vi "Verify Font availability.vi"(0 "Font IN":refnum<class "Font Class.lvclass">, 7 "Font name":string, 9 "One button message (F)?":bool, 11 "error in (no error)":errorcluster) -> (4 "Font duplicate":refnum<class "Font Class.lvclass">, 8 "Font":string, 15 "error out":errorcluster)   [LabVIEW 2019, in "Exaprom PDF.lvlib" / "Font Class.lvclass"]
doc: "Version 1.0\nDeveloped by Jean-Marc Simard\nCopyright © 2010, Exaprom Inc.\nAll rights reserved.\nLicense: BSD\n\nWith iTextSharp 4.1.6 (http://itextsharp.sourceforge.net)\nunder Mozilla Public License Version 1.1\n(http://www.mozilla.org/MPL/MPL-1.1.html)"
uses:
  Font Class.lvclass
  Font Class.lvclass/Font Class.ctl
  Exaprom PDF.lvlib
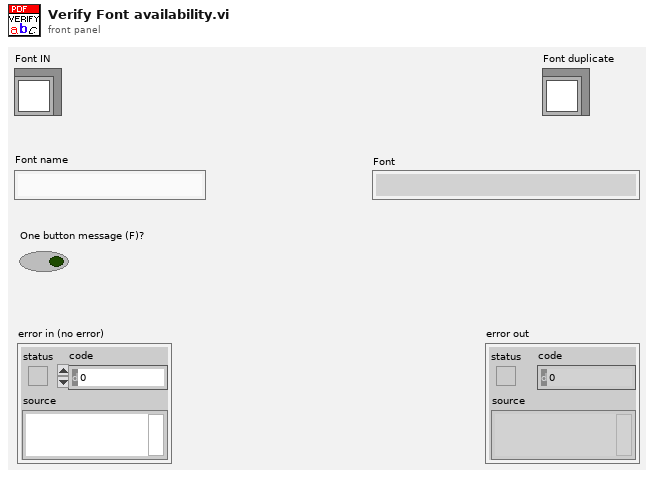
[diagram p1: front panel]
types:
  T1 = cluster{"Font name":string, "File name":string}[]
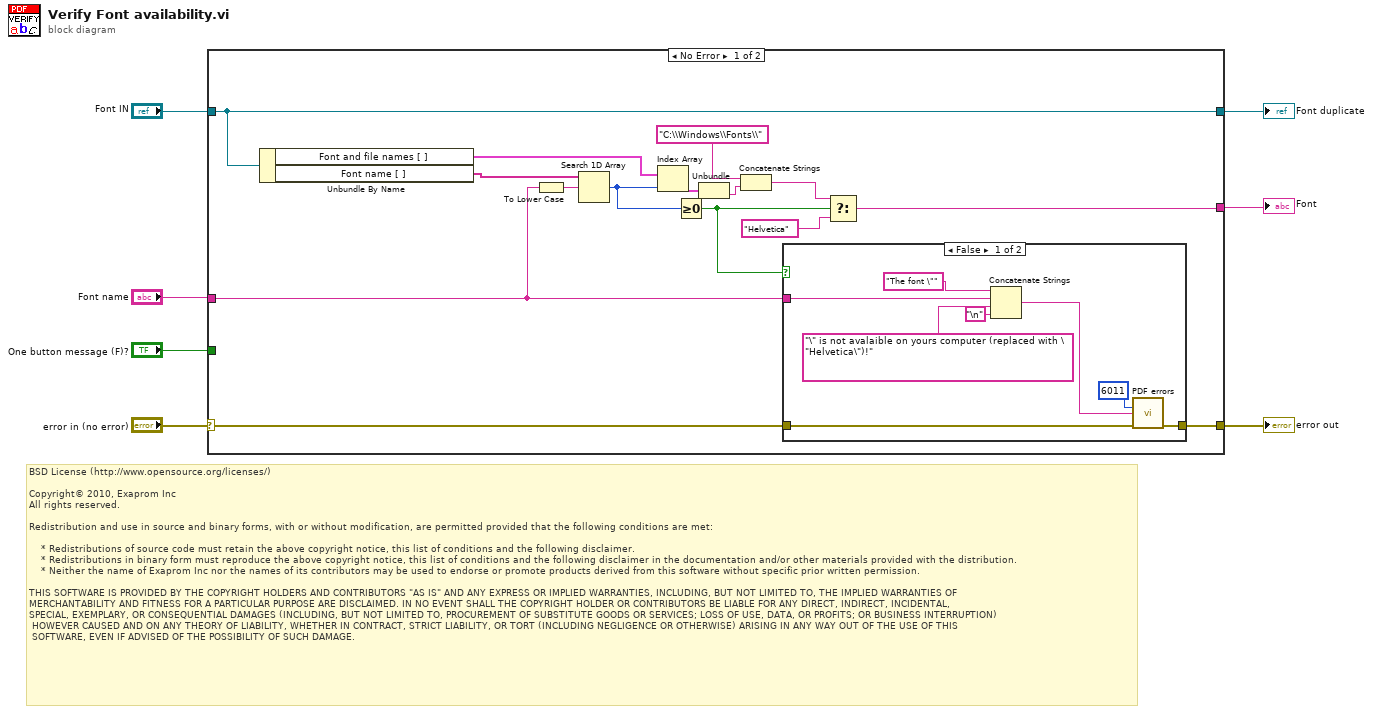
[diagram p0: block diagram]
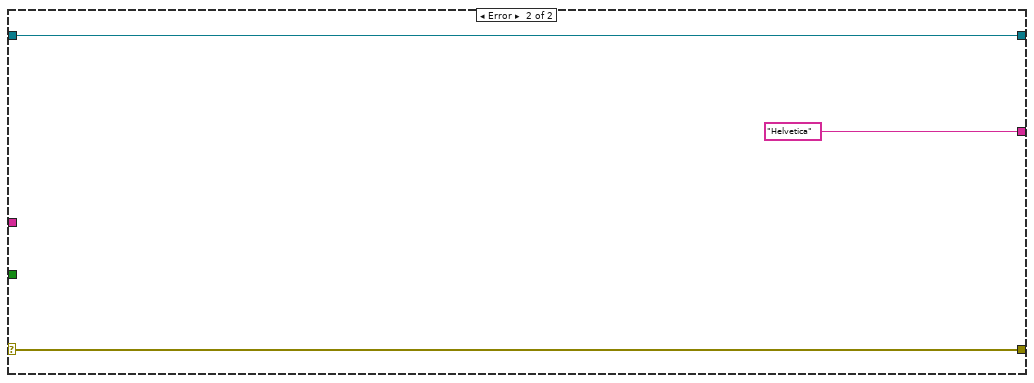
[diagram p3: hidden frame]
diagram:
  # "BSD License (http://www.opensource.org/licenses/)\n\nCopyright© 2010, Exaprom Inc\nAll rights reserved.\n\nRedistribution and use in source and binary forms, with or without modification, are permitted provided that the following conditions are met:\n\n    * Redistributions of source code must retain the above copyright notice, this list of conditions and the following disclaimer.\n    * Redistributions in binary form must reproduce the above copyright notice, this list of conditions and the following disclaimer in the documentation and/or other materials provided with the distribution.\n    * Neither the name of Exaprom Inc nor the names of its contributors may be used to endorse or promote products derived from this software without specific prior written permission.\n\nTHIS SOFTWARE IS PROVIDED BY THE COPYRIGHT HOLDERS AND CONTRIBUTORS \"AS IS\" AND ANY EXPRESS OR IMPLIED WARRANTIES, INCLUDING, BUT NOT LIMITED TO, THE IMPLIED WARRANTIES OF \nMERCHANTABILITY AND FITNESS FOR A PARTICULAR PURPOSE ARE DISCLAIMED. IN NO EVENT SHALL THE COPYRIGHT HOLDER OR CONTRIBUTORS BE LIABLE FOR ANY DIRECT, INDIRECT, INCIDENTAL,\nSPECIAL, EXEMPLARY, OR CONSEQUENTIAL DAMAGES (INCLUDING, BUT NOT LIMITED TO, PROCUREMENT OF SUBSTITUTE GOODS OR SERVICES; LOSS OF USE, DATA, OR PROFITS; OR BUSINESS INTERRUPTION)\n HOWEVER CAUSED AND ON ANY THEORY OF LIABILITY, WHETHER IN CONTRACT, STRICT LIABILITY, OR TORT (INCLUDING NEGLIGENCE OR OTHERWISE) ARISING IN ANY WAY OUT OF THE USE OF THIS\n SOFTWARE, EVEN IF ADVISED OF THE POSSIBILITY OF SUCH DAMAGE."
  n1 = case shown="No Error" "error in (no error)" {
    selector: "error in (no error)" -> [w11 w34]
    tunnel: [w12 w34] -> w7
    tunnel: [w15 "Helvetica"] -> w5
    tunnel: "Font name" -> [w14 _]
    tunnel: "One button message (F)?" -> [_ _]
    tunnel: "Font IN" -> [w8 w32]
    tunnel: [w8 w32] -> w1
    frame No Error {
      n2 = Unbundle By Name(w8) -> ("Font and file names [ ]"=w10:T1, "Font name [ ]"=w9:string[])
      n3 = To Lower Case(string=w14) -> (all lower case string=w22:string)
      n4 = Search 1D Array(1D array=w9, element=w22) -> (index of element=w19:i32)  [unwired: 1 out]
      n5 = Index Array(array=w10, index=w19) -> (element=w17:cluster{"Font name":string, "File name":string})
      n6 = Greater Or Equal To 0?(x=w19) -> (x >= 0?=w13:bool)
      n7 = Unbundle(w17) -> ("File name"=w18:string)  [unwired: 1 out]
      n8 = Concatenate Strings("C:\\Windows\\Fonts\\", w18) -> (w20:string)
      n9 = case shown="False" w13 {
        tunnel: w14 -> [w29 _]
        tunnel: [w26 w31] -> w12
        tunnel: w11 -> [w25 w31]
        frame False {
          n10 = Concatenate Strings("The font \"", w29, "\" is not avalaible on yours computer (replaced with \"Helvetica\")!" ("string"), "\n") -> (w24:string)
          n11 = call "PDF errors.vi"("code"=6011, "Additionnal information"=w24, "error in (no error)"=w25) -> ("error out"=w26:errorcluster)  [unwired: 12 out]
        }
        frame True {
        }
      }
      n12 = Select(t=w20, s=w13, f="Helvetica") -> (s? t:f=w15:string)
    }
    frame Error {
    }
  }
  "error out" <- w7
  "Font" <- w5
  "Font duplicate" <- w1
